vi "弹窗-指定网卡本机IP选择.vi"(11 "IP地址[]":string[](array[string])) -> (3 "选择的IP":string)   [LabVIEW 2017]
panel:
  in  "本机IP枚举":u16(ring) caption="本机IP地址" items=["192.168.1.150", "10.1.79.57"]
  in  "确定":bool
  in  "取消":bool
  out "信号-结束事件结构":bool=TRUE
  # "选择指定网卡下的本机地址\n或者断开其他网络"
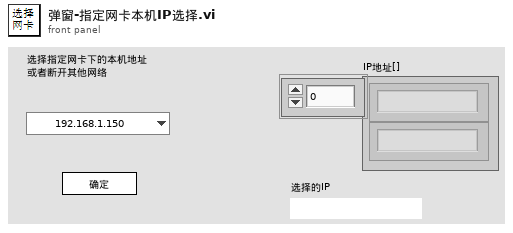
[diagram p1: front panel]
types:
  T1 = enum32{"Invalid", "Standard", "Closed", "Hidden", "Minimized", "Maximized"}
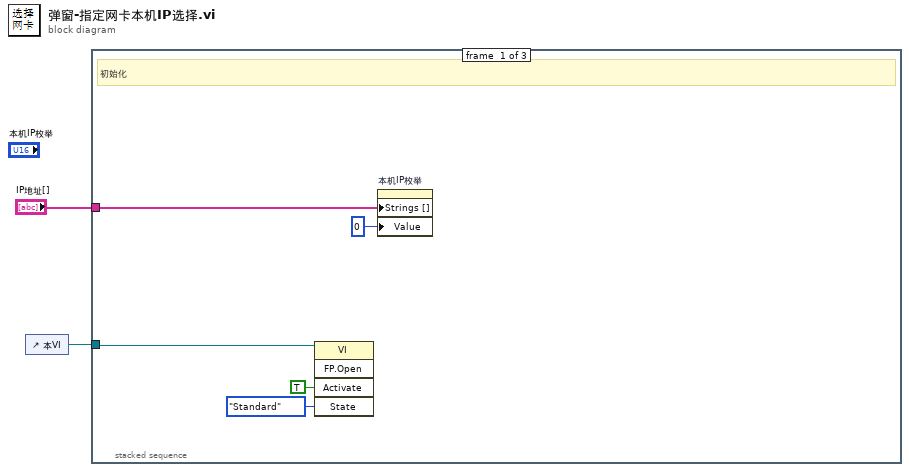
[diagram p0: block diagram]
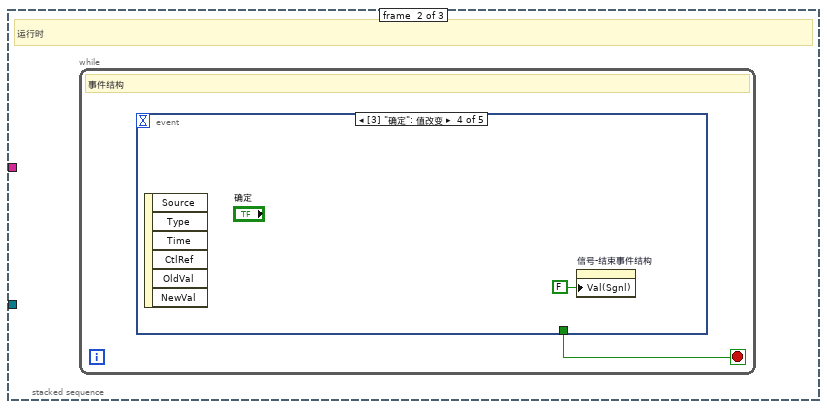
[diagram p2: hidden frame]
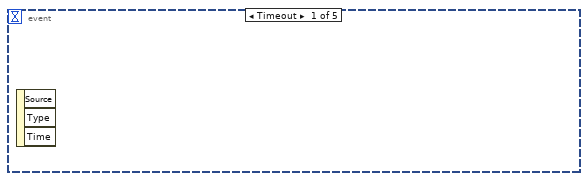
[diagram p3: hidden frame]
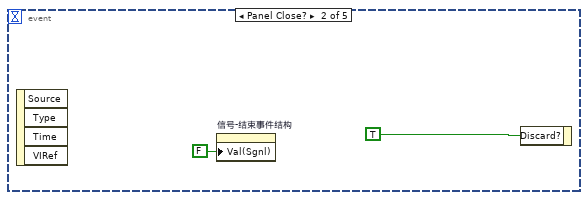
[diagram p4: hidden frame]
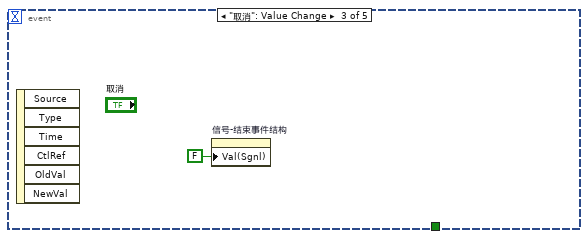
[diagram p5: hidden frame]
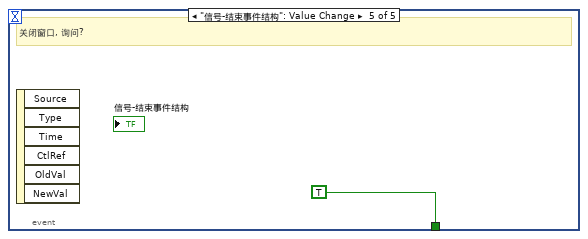
[diagram p6: hidden frame]
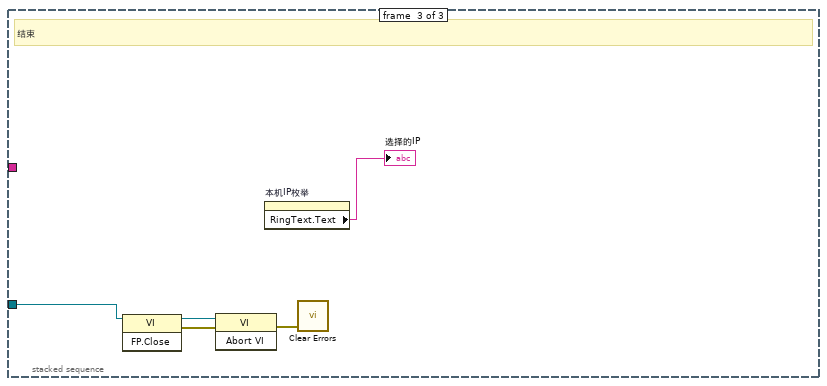
[diagram p7: hidden frame]
diagram:
  n1 = control-ref of="本VI"() -> (w2:refnum<vi>)
  n2 = stacked-sequence {
    tunnel: w2 -> [w7 _ w18]
    tunnel: "IP地址[]" -> [w4 _ _]
    frame #0 {
      # "初始化"
      n3 = invoke class="VI" method="FP.Open"(reference=w7, "Activate"=TRUE ("激活？"), "State"=T1."Standard" ("状态")) -> ()  [unwired: 2 in, 5 out]
      n4 = property on="本机IP枚举" class="Ring (严格)"("Strings []"=w4, "Value"=0) -> ()  [unwired: 2 in, 2 out]
    }
    frame #1 {
      # "运行时"
      n5 = while {
        stop <- w8 stop-if-true
        # "事件结构"
        n6 = event shown="[3] \"确定\": 值改变" {
          selector: _ -> [_ _ _ _ _]
          dyn-events: _ -> [_ _ _ _ _]
          timeout: _ -> [_ _ _ _ _]
          tunnel: [_ _ _ _ TRUE] -> w8
          event Timeout {
            n7 = event-data() -> ()  [unwired: 1 in, 3 out]
          }
          event Panel Close? {
            n8 = event-data() -> ()  [unwired: 1 in, 4 out]
            n9 = property on="信号-结束事件结构" class="Bool (严格)"("Val(Sgnl)"=FALSE ("值(信号)")) -> ()  [unwired: 2 in, 2 out]
            n10 = event-data("Discard?"=TRUE ("放弃？")) -> ()  [unwired: 1 in, 1 out]
          }
          event "取消": Value Change {
            n11 = event-data() -> ()  [unwired: 1 in, 6 out]
            n12 = property on="信号-结束事件结构" class="Bool (严格)"("Val(Sgnl)"=FALSE ("值(信号)")) -> ()  [unwired: 2 in, 2 out]
          }
          event "确定": Value Change {
            n13 = event-data() -> ()  [unwired: 1 in, 6 out]
            n14 = property on="信号-结束事件结构" class="Bool (严格)"("Val(Sgnl)"=FALSE ("值(信号)")) -> ()  [unwired: 2 in, 2 out]
          }
          event "信号-结束事件结构": Value Change {
            # "关闭窗口, 询问?"
            n15 = event-data() -> ()  [unwired: 1 in, 6 out]
          }
        }
      }
    }
    frame #2 {
      # "结束"
      n16 = invoke class="VI" method="FP.Close"(reference=w18) -> (reference out=w17:refnum<vi>, error out=w16:errorcluster)  [unwired: 2 in, 1 out]
      n17 = invoke class="VI" method="Abort VI"(reference=w17, error in=w16) -> (error out=w15:errorcluster)  [unwired: 1 in, 2 out]
      n18 = property on="本机IP枚举" class="Ring (严格)"() -> ("RingText.Text"=→"选择的IP":string)  [unwired: 2 in, 2 out]
      n19 = call <vilib>:"Clear Errors.vi"("error in (no error)"=w15) -> ()  [unwired: 5 in, 2 out]
    }
  }
